vi "LaserCal-Restore Defaults.vi"() -> (8 "Settings":T1={"System ID"={"Name"="", "Laser SN"="", "Wavelength (nm)"=473.0, "Fiber diameter (um)"=400.0, "Power setting"=100.0}, "Sensor"={"Average (ms)"=100.0, "Range"="140mW"}, "Meter"={"Vcommand"=0.0, "scale"=enum."linear", "Pulsed"=FALSE, "Pulse width (ms)"=0.0, "Pulse rate (Hz)"=0.0, "mode"=enum."Voltage only"}, "Static"={"Stimulus"={"scale"=enum."linear", "Voltage"="0:0.5:5"}, "Response"={"Settle time (s)"=1.0, "Tmeasure (s)"=2.0}}, "Pulsed"={"Stimulus"={"Vcommand Expr"="0:0.5:5", "Width Expr"="10", "mode"=enum."Voltage only", "Rate Expr"="50", "randomize"=TRUE}, "Response"={"Settle time (s)"=1.0, "Tmeasure (s)"=2.0, "Repeats"=2}}, "Options"={"current"=FALSE, "save current"=FALSE, "mA/V"=0.0}})   [LabVIEW 2015]
uses:
  Typedefs/LaserCal-Settings.ctl
  Typedefs/LaserCal-System ID.ctl
  Typedefs/LaserCal-Meter Stimulus.ctl
  Typedefs/LaserCal-Control Mode.ctl
  Typedefs/LaserCal-IO Stimulus Params.ctl
  Typedefs/LaserCal-IO Response Params.ctl
  Typedefs/LaserCal-Stimulus Params.ctl
  Typedefs/LaserCal-Response (PT).ctl
  Typedefs/LaserCal-Options.ctl
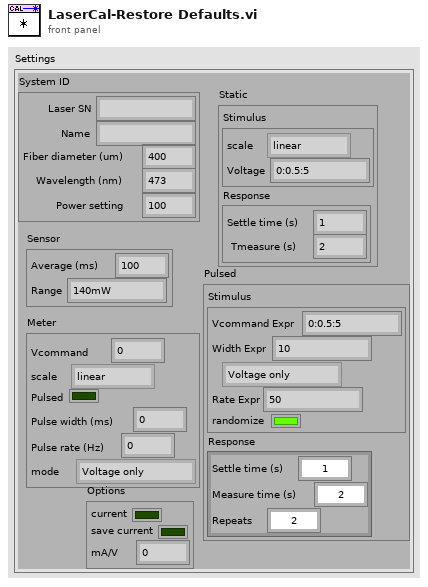
[diagram p1: front panel]
types:
  T1 = typedef "LaserCal-Settings.ctl" = cluster{"System ID":T2, "Sensor":cluster{"Average (ms)":dbl, "Range":string}, "Meter":T3, "Static":cluster{"Stimulus":T5, "Response":T6}, "Pulsed":cluster{"Stimulus":T7, "Response":T8}, "Options":T9}
  T2 = typedef "LaserCal-System ID.ctl" = cluster{"Name":string, "Laser SN":string, "Wavelength (nm)":dbl, "Fiber diameter (um)":dbl, "Power setting":dbl}
  T3 = typedef "LaserCal-Meter Stimulus.ctl" = cluster{"Vcommand":dbl, "scale":enum16{"linear", "dB"}, "Pulsed":bool, "Pulse width (ms)":dbl, "Pulse rate (Hz)":dbl, "mode":T4}
  T4 = typedef "LaserCal-Control Mode.ctl" = enum16{"Voltage only", "Voltage + Enable"}
  T5 = typedef "LaserCal-IO Stimulus Params.ctl" = cluster{"scale":enum16{"linear", "dB"}, "Voltage":string}
  T6 = typedef "LaserCal-IO Response Params.ctl" = cluster{"Settle time (s)":dbl, "Tmeasure (s)":dbl}
  T7 = typedef "LaserCal-Stimulus Params.ctl" = cluster{"Vcommand Expr":string, "Width Expr":string, "mode":T4, "Rate Expr":string, "randomize":bool}
  T8 = typedef "LaserCal-Response (PT).ctl" = cluster{"Settle time (s)":dbl, "Tmeasure (s)":dbl, "Repeats":i32}
  T9 = typedef "LaserCal-Options.ctl" = cluster{"current":bool, "save current":bool, "mA/V":dbl}
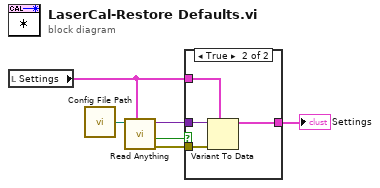
[diagram p0: block diagram]
diagram:
  n1 = local read "Settings"() -> (w2:T1)
  n2 = call "Config File Path.vi"() -> ("Default config file name"=w6:path)  [unwired: 1 in]
  n3 = call "Read Anything.vi"("Type of Anything"=w2, "Path (dialog)"=w6) -> ("Error Out"=w4:errorcluster, "Found?"=w5:bool, "Anything"=w3:variant)  [unwired: 7 in]
  n4 = case shown="True" w5 {
    tunnel: w4 -> [_ w11]
    tunnel: w3 -> [_ w10]
    tunnel: w2 -> [w7 w9]
    tunnel: [w7 w8] -> w1
    frame False {
    }
    frame True {
      n5 = Variant To Data(error in=w11, type=w9, Variant=w10) -> (data=w8:T1)  [unwired: 1 out]
    }
  }
  "Settings" <- w1
